vi "espectroMOKE.vi"() -> ()   [LabVIEW 2016]
uses:
  <vilib>/Utility/file.llb/Write Delimited Spreadsheet (DBL).vi
panel:
  in  "Nombre (guardar como .txt)":path
  in  "stop":bool
  in  "PEM_VISA":refnum<visa-resource-name>="COM6"
  in  "monocromador":refnum<visa-resource-name>="COM3"
  in  "Tab Control":enum32{"medicion", "configuracion"}(tab)=enum."configuracion"
  in  "inicio":bool
  out "longitud  onda":dbl
  in  "lecturas":i32
  out "UpMult":dbl
  out "UpLockin":dbl
  in  "Paso":dbl
  in  "Fin":dbl
  in  "Inicio":dbl
  out "division":cluster{"array":dbl[], "array":dbl[]}(graph)
  out "multimetro":cluster{"array":dbl[], "array":dbl[]}(graph)
  out "Lock_In":cluster{"array":dbl[], "array":dbl[]}(graph)
  in  "PEM":bool=TRUE
  out "lamda":dbl=600.0
  in  "Longitud de onda":dbl=600.0
  in  "monocrom":bool
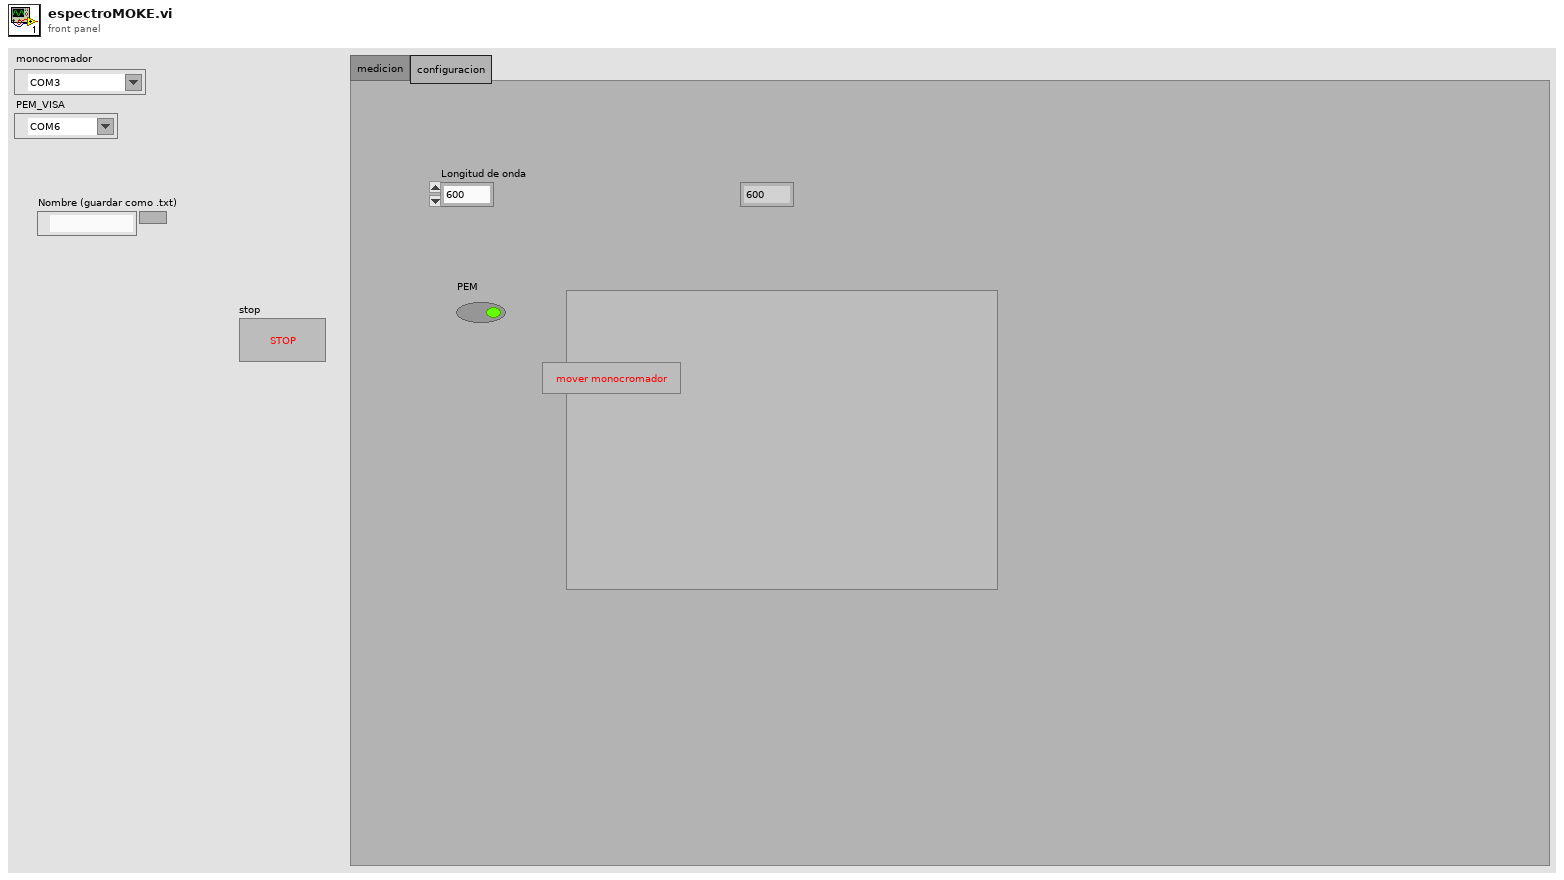
[diagram p1: front panel]
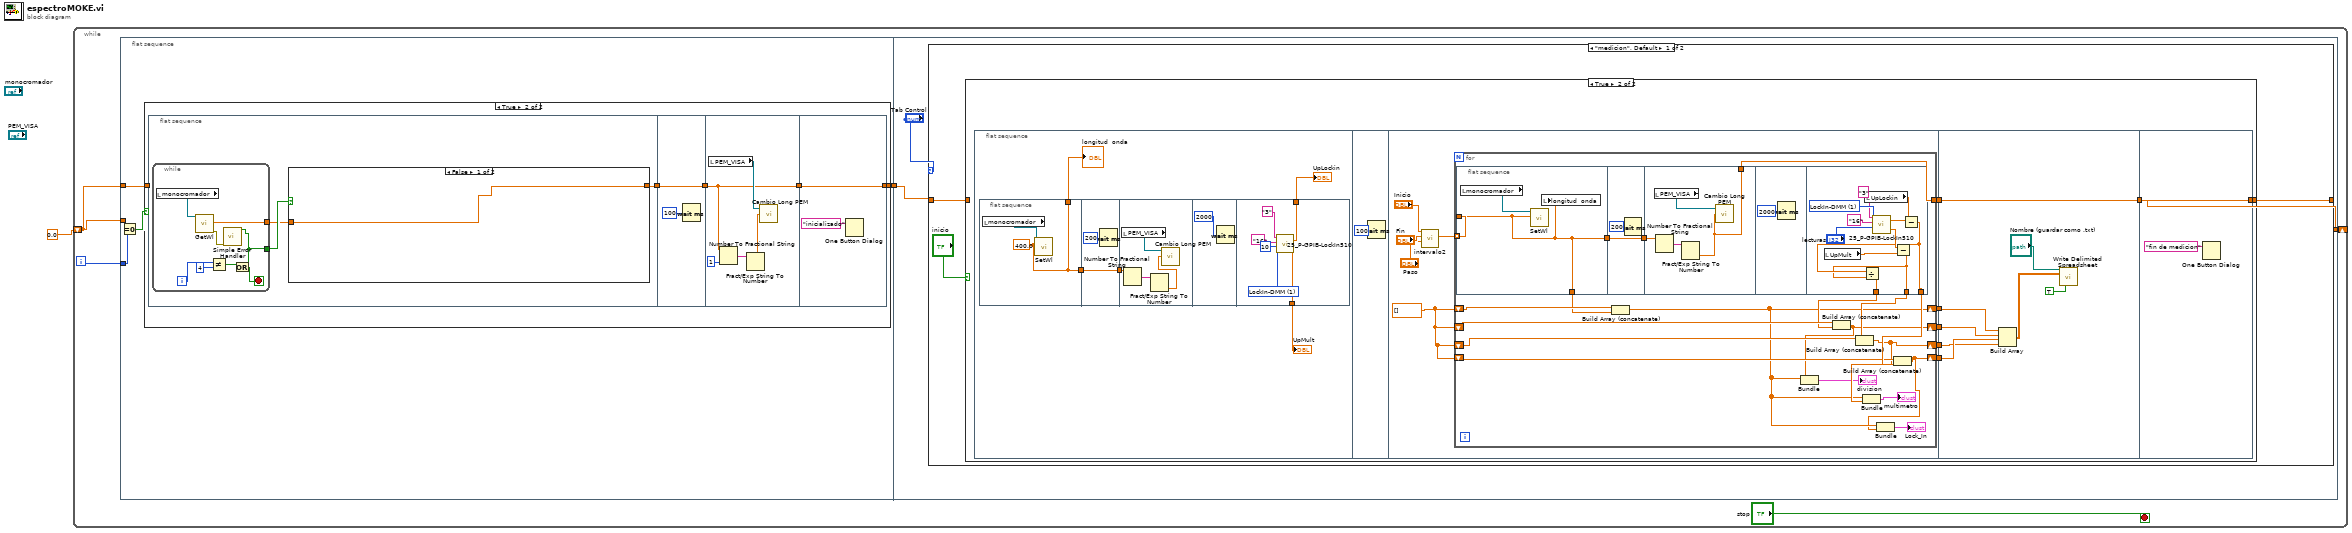
[diagram p0: block diagram]
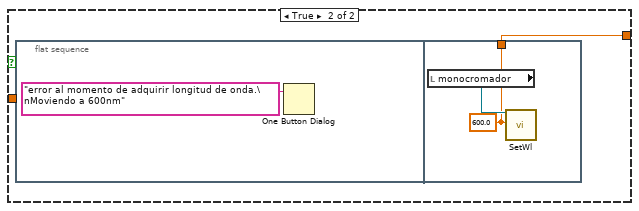
[diagram p3: hidden frame]
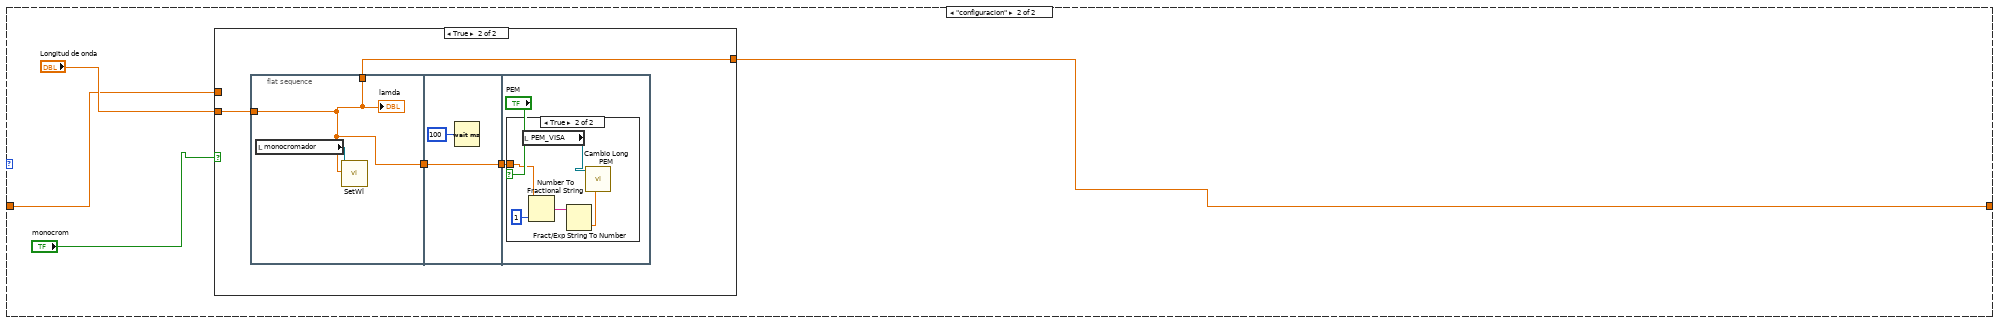
[diagram p5: hidden frame]
diagram:
  n1 = while {
    shift-right: [w3] -> _
    shift-left: 0.0 -> [w6]
    i -> [w5]
    stop <- "stop" stop-if-true
    n2 = flat-sequence {
      tunnel: w6 -> [w10]
      tunnel: w6 -> [_]
      tunnel: w5 -> [w9]
      tunnel: [w7] -> w4
      tunnel: w4 -> [w42]
      tunnel: [w41] -> w3
      frame #0 {
        n3 = Equal To 0?(x=w9) -> (x = 0?=w8:bool)
        n4 = case shown="True" w8 {
          tunnel: [w11 w15] -> w7
          tunnel: w10 -> [w11 _]
          frame False {
          }
          frame True {
            n5 = flat-sequence {
              tunnel: [w16] -> w14
              tunnel: w14 -> [w33]
              tunnel: [w33] -> w13
              tunnel: w13 -> [w37]
              tunnel: [w37] -> w12
              tunnel: [w40] -> w15
              tunnel: w12 -> [w40]
              frame #0 {
                n6 = while {
                  tunnel: [w26] -> w17
                  tunnel: [w25] -> w18
                  i -> [w31]
                  stop <- w28 stop-if-true
                  n7 = local read "monocromador"() -> (w24:refnum<visa-resource-name>)
                  n8 = call "GetWl.vi"("VISA resource name"=w24) -> ("Wavelength"=w26:dbl, "error out"=w27:errorcluster)  [unwired: 16 in, 1 out]
                  n9 = Not Equal?(x=w31, y=4) -> (x != y?=w29:bool)
                  n10 = call <vilib>:"Simple Error Handler.vi"("error in (no error)"=w27) -> ("error?"=w25:bool)  [unwired: 4 in, 4 out]
                  n11 = Or(x=w29, y=w25) -> (x .or. y?=w28:bool)
                }
                n12 = case shown="False" w18 {
                  tunnel: w17 -> [w19 _]
                  tunnel: [w19 w20] -> w16
                  frame False {
                  }
                  frame True {
                    n13 = flat-sequence {
                      tunnel: [w22] -> w20
                      frame #0 {
                        n14 = One Button Dialog(message="error al momento de adquirir longitud de onda.\nMoviendo a 600nm") -> ()  [unwired: 1 in, 1 out]
                      }
                      frame #1 {
                        w22 = sgl 600.0 ("Wavelength (nm)")
                        n15 = local read "monocromador"() -> (w23:refnum<visa-resource-name>)
                        n16 = call "SetWl.vi"("VISA resource name"=w23, "Wavelength (nm)"=w22) -> ()  [unwired: 16 in, 2 out]
                      }
                    }
                  }
                }
              }
              frame #1 {
                n17 = Wait (ms)(milliseconds to wait=u32 100) -> ()  [unwired: 1 out]
              }
              frame #2 {
                n18 = local read "PEM_VISA"() -> (w38:refnum<visa-resource-name>)
                n19 = Number To Fractional String(number=w37, precision (6)=i16 1) -> (F-format string=w36:string)  [unwired: 2 in]
                n20 = Fract/Exp String To Number(string=w36) -> (number=w34:dbl)  [unwired: 3 in, 1 out]
                n21 = call "Cambio Long PEM.vi"("Long de Onda"=w34, "VISA Refnum in"=w38) -> ()  [unwired: 1 in, 2 out]
              }
              frame #3 {
                n22 = One Button Dialog(message="inicializado") -> ()  [unwired: 1 in, 1 out]
              }
            }
          }
        }
      }
      frame #1 {
        n23 = case shown="\"medicion\", Default" "Tab Control" {
          tunnel: w42 -> [w45 w135]
          tunnel: [w46 w136] -> w41
          frame "medicion", Default {
            n24 = case shown="True" "inicio" {
              tunnel: [w47 w49] -> w46
              tunnel: w45 -> [w47 _]
              frame False {
              }
              frame True {
                n25 = flat-sequence {
                  tunnel: [w80] -> w54
                  tunnel: [w79] -> w53
                  tunnel: [w78] -> w52
                  tunnel: [w77] -> w51
                  tunnel: [w76] -> w50
                  tunnel: w54 -> [w132]
                  tunnel: w53 -> [w130]
                  tunnel: w52 -> [w129]
                  tunnel: w51 -> [w128]
                  tunnel: w50 -> [w127]
                  tunnel: [w132] -> w48
                  tunnel: [w134] -> w49
                  tunnel: w48 -> [w134]
                  frame #0 {
                    n26 = flat-sequence {
                      tunnel: [w60] -> w59
                      tunnel: [w60] -> w55
                      tunnel: w59 -> [w62]
                      tunnel: [w62] -> w58
                      tunnel: w58 -> [w67]
                      tunnel: [w70] -> w57
                      tunnel: [w69] -> w56
                      frame #0 {
                        w60 = sgl 400.0 ("Wavelength (nm)")
                        n27 = local read "monocromador"() -> (w61:refnum<visa-resource-name>)
                        n28 = call "SetWl.vi"("VISA resource name"=w61, "Wavelength (nm)"=w60) -> ()  [unwired: 16 in, 2 out]
                      }
                      frame #1 {
                        n29 = Wait (ms)(milliseconds to wait=u32 200) -> ()  [unwired: 1 out]
                      }
                      frame #2 {
                        n30 = local read "PEM_VISA"() -> (w64:refnum<visa-resource-name>)
                        n31 = Number To Fractional String(number=w67) -> (F-format string=w66:string)  [unwired: 3 in]
                        n32 = Fract/Exp String To Number(string=w66) -> (number=w65:dbl)  [unwired: 3 in, 1 out]
                        n33 = call "Cambio Long PEM.vi"("Long de Onda"=w65, "VISA Refnum in"=w64) -> ()  [unwired: 1 in, 2 out]
                      }
                      frame #3 {
                        n34 = Wait (ms)(milliseconds to wait=u32 2000) -> ()  [unwired: 1 out]
                      }
                      frame #4 {
                        w72 = u16 1 items=["LockIn", "LockIn-DMM"] ("Tipo")
                        n35 = call "25_P-GPIB-LockIn510.vi"("Tipo"=w72, "Lecturas"=10, "P-DMM"="16", "P-LockIn"="3") -> ("DMM"=w70:dbl, "LockIn"=w69:dbl)
                      }
                    }
                    "longitud  onda" <- w55
                    "UpMult" <- w57
                    "UpLockin" <- w56
                  }
                  frame #1 {
                    n36 = Wait (ms)(milliseconds to wait=u32 100) -> ()  [unwired: 1 out]
                  }
                  frame #2 {
                    w81 = dbl[] []
                    n37 = call "intervalo2.vi"("incremento"="Paso", "fin"="Fin", "inicio"="Inicio") -> ("Array"=w85:dbl[])  [unwired: 8 in]
                    n38 = for {
                      tunnel: w85 -> [w104] mode=indexing
                      shift-right: [w88] -> w79
                      shift-left: w81 -> [w101]
                      shift-right: [w93] -> w78
                      shift-left: w81 -> [w99]
                      shift-right: [w91] -> w76
                      shift-left: w81 -> [w97]
                      shift-right: [w87] -> w77
                      shift-left: w81 -> [w94]
                      tunnel: [w86] -> w80
                      n39 = flat-sequence {
                        tunnel: w104 -> [w105]
                        tunnel: [w105] -> w103
                        tunnel: [w105] -> w100
                        tunnel: w103 -> [w107]
                        tunnel: [w107] -> w102
                        tunnel: w102 -> [w112]
                        tunnel: [w109] -> w86
                        tunnel: [w115] -> w95
                        tunnel: [w114] -> w96
                        tunnel: [w116] -> w98
                        frame #0 {
                          n40 = local read "monocromador"() -> (w106:refnum<visa-resource-name>)
                          n41 = call "SetWl.vi"("VISA resource name"=w106, "Wavelength (nm)"=w105) -> ()  [unwired: 16 in, 2 out]
                          n42 = local write "longitud  onda"(w105) -> ()
                        }
                        frame #1 {
                          n43 = Wait (ms)(milliseconds to wait=u32 200) -> ()  [unwired: 1 out]
                        }
                        frame #2 {
                          n44 = local read "PEM_VISA"() -> (w110:refnum<visa-resource-name>)
                          n45 = Number To Fractional String(number=w112) -> (F-format string=w111:string)  [unwired: 3 in]
                          n46 = Fract/Exp String To Number(string=w111) -> (number=w109:dbl)  [unwired: 3 in, 1 out]
                          n47 = call "Cambio Long PEM.vi"("Long de Onda"=w109, "VISA Refnum in"=w110) -> ()  [unwired: 1 in, 2 out]
                        }
                        frame #3 {
                          n48 = Wait (ms)(milliseconds to wait=u32 2000) -> ()  [unwired: 1 out]
                        }
                        frame #4 {
                          w123 = u16 1 items=["LockIn", "LockIn-DMM"] ("Tipo")
                          n49 = local read "UpMult"() -> (w117:dbl)
                          n50 = local read "UpLockin"() -> (w119:dbl)
                          n51 = call "25_P-GPIB-LockIn510.vi"("Tipo"=w123, "Lecturas"="lecturas", "P-DMM"="16", "P-LockIn"="3") -> ("DMM"=w118:dbl, "LockIn"=w120:dbl)
                          n52 = Subtract(x=w118, y=w117) -> (x-y=w114:dbl)
                          n53 = Subtract(x=w120, y=w119) -> (x-y=w115:dbl)
                          n54 = Divide(x=w115, y=w114) -> (x/y=w116:dbl)
                        }
                      }
                      n55 = Build Array (concatenate)(w101, w100) -> (w88:dbl[])
                      n56 = Build Array (concatenate)(w99, w98) -> (w93:dbl[])
                      n57 = Bundle(w88, w93) -> (→"division":cluster{dbl[], dbl[]})  [unwired: 1 in]
                      n58 = Build Array (concatenate)(w97, w96) -> (w91:dbl[])
                      n59 = Bundle(w88, w91) -> (→"multimetro":cluster{dbl[], dbl[]})  [unwired: 1 in]
                      n60 = Build Array (concatenate)(w94, w95) -> (w87:dbl[])
                      n61 = Bundle(w88, w87) -> (→"Lock_In":cluster{dbl[], dbl[]})  [unwired: 1 in]
                    }
                  }
                  frame #3 {
                    n62 = Build Array(w130, w129, w128, w127) -> (w131:dbl[][])
                    n63 = call-poly <vilib>:"Write Delimited Spreadsheet.vi"("file path (dialog if empty)"="Nombre (guardar como .txt)", "2D data"=w131, "transpose? (no:F)"=TRUE) -> ()  [unwired: 11 in, 2 out]
                  }
                  frame #4 {
                    n64 = One Button Dialog(message="fin de medicion") -> ()  [unwired: 1 in, 1 out]
                  }
                }
              }
            }
          }
          frame "configuracion" {
            n65 = case shown="True" "monocrom" {
              tunnel: "Longitud de onda" -> [_ w143]
              tunnel: [w139 w142] -> w136
              tunnel: w135 -> [w139 _]
              frame False {
              }
              frame True {
                n66 = flat-sequence {
                  tunnel: w143 -> [w144]
                  tunnel: [w144] -> w141
                  tunnel: [w144] -> w142
                  tunnel: w141 -> [w147]
                  tunnel: [w147] -> w140
                  tunnel: w140 -> [w148]
                  frame #0 {
                    n67 = local read "monocromador"() -> (w145:refnum<visa-resource-name>)
                    n68 = call "SetWl.vi"("VISA resource name"=w145, "Wavelength (nm)"=w144) -> ()  [unwired: 16 in, 2 out]
                    "lamda" <- w144
                  }
                  frame #1 {
                    n69 = Wait (ms)(milliseconds to wait=u32 100) -> ()  [unwired: 1 out]
                  }
                  frame #2 {
                    n70 = case shown="True" "PEM" {
                      tunnel: w148 -> [_ w151]
                      frame False {
                      }
                      frame True {
                        n71 = local read "PEM_VISA"() -> (w154:refnum<visa-resource-name>)
                        n72 = Number To Fractional String(number=w151, precision (6)=i16 1) -> (F-format string=w153:string)  [unwired: 2 in]
                        n73 = Fract/Exp String To Number(string=w153) -> (number=w150:dbl)  [unwired: 3 in, 1 out]
                        n74 = call "Cambio Long PEM.vi"("Long de Onda"=w150, "VISA Refnum in"=w154) -> ()  [unwired: 1 in, 2 out]
                      }
                    }
                  }
                }
              }
            }
          }
        }
      }
    }
  }
